vi "sensor model (SubVI).vi"(0 "Sensor noise":bool, 1 "nu in":dbl[](array[numeric])=[-0.0018015758017567245, -0.001192557883344063, -0.016303156939595005, 0.0001609866843798056, -3.986241544768407e-05, 0.002433779794769443], 2 "std HiPAP":dbl=0.1, 3 "Sample period HiPAP":dbl=1000.0, 4 "std IMU":dbl=0.02, 5 "eta in":dbl[](array[numeric])=[0.004584023716384989, -0.00136654983894139, 20.08049813655914, 1.4271590869671887e-05, -0.00011626978763392943, 1.5737394787921046], 6 "Init North":dbl=6971450.0 format="%#.2f", 7 "All Pos mes":bool, 8 "std rad/s":dbl=0.02, 9 "std PG":dbl=0.1, 10 "Seafloor":dbl[](array[numeric])=[30.0, -0.1, 0.0, 0.0, 0.0], 11 "Init East":dbl=395890.0 format="%#.2f", 12 "std DVL":dbl=0.1, 13 "NORTH SHIP":dbl=7100000.0, 14 "HEADING SHIP":dbl=488000.0, 15 "EAST SHIP":dbl=488000.0, 16 "Init Depth":dbl=4.0 format="%#.2f", 17 "std roll&pitch":dbl=0.02) -> (19 "GPS and APOS Strings":string[](array[string]), 20 "COM1":dbl[](array[numeric])=[20.08041093421861, 29.91885735344196, 0.0, 90.0, 2068.0], 23 "COM2":dbl[](array[numeric])=[539999.2486367036, 7200000.006791385, -0.0030178927294211453, -0.0018015758017567245, 12.750414264450102, -85.11865540641482, 20.696406625105084, 54.45747480595215])   [LabVIEW 2014]
uses:
  <vilib>/Analysis/NI_AALBase.lvlib
panel:
  out "Heave":cluster{"Y":dbl[], "Y":dbl[]}[](graph)
  out "Surge":cluster{"Y":dbl[], "Y":dbl[]}[](graph)
  out "Sway":cluster{"Y":dbl[], "Y":dbl[]}[](graph)
  out "PSIMSSB String":string
  out "GPGGA String":string
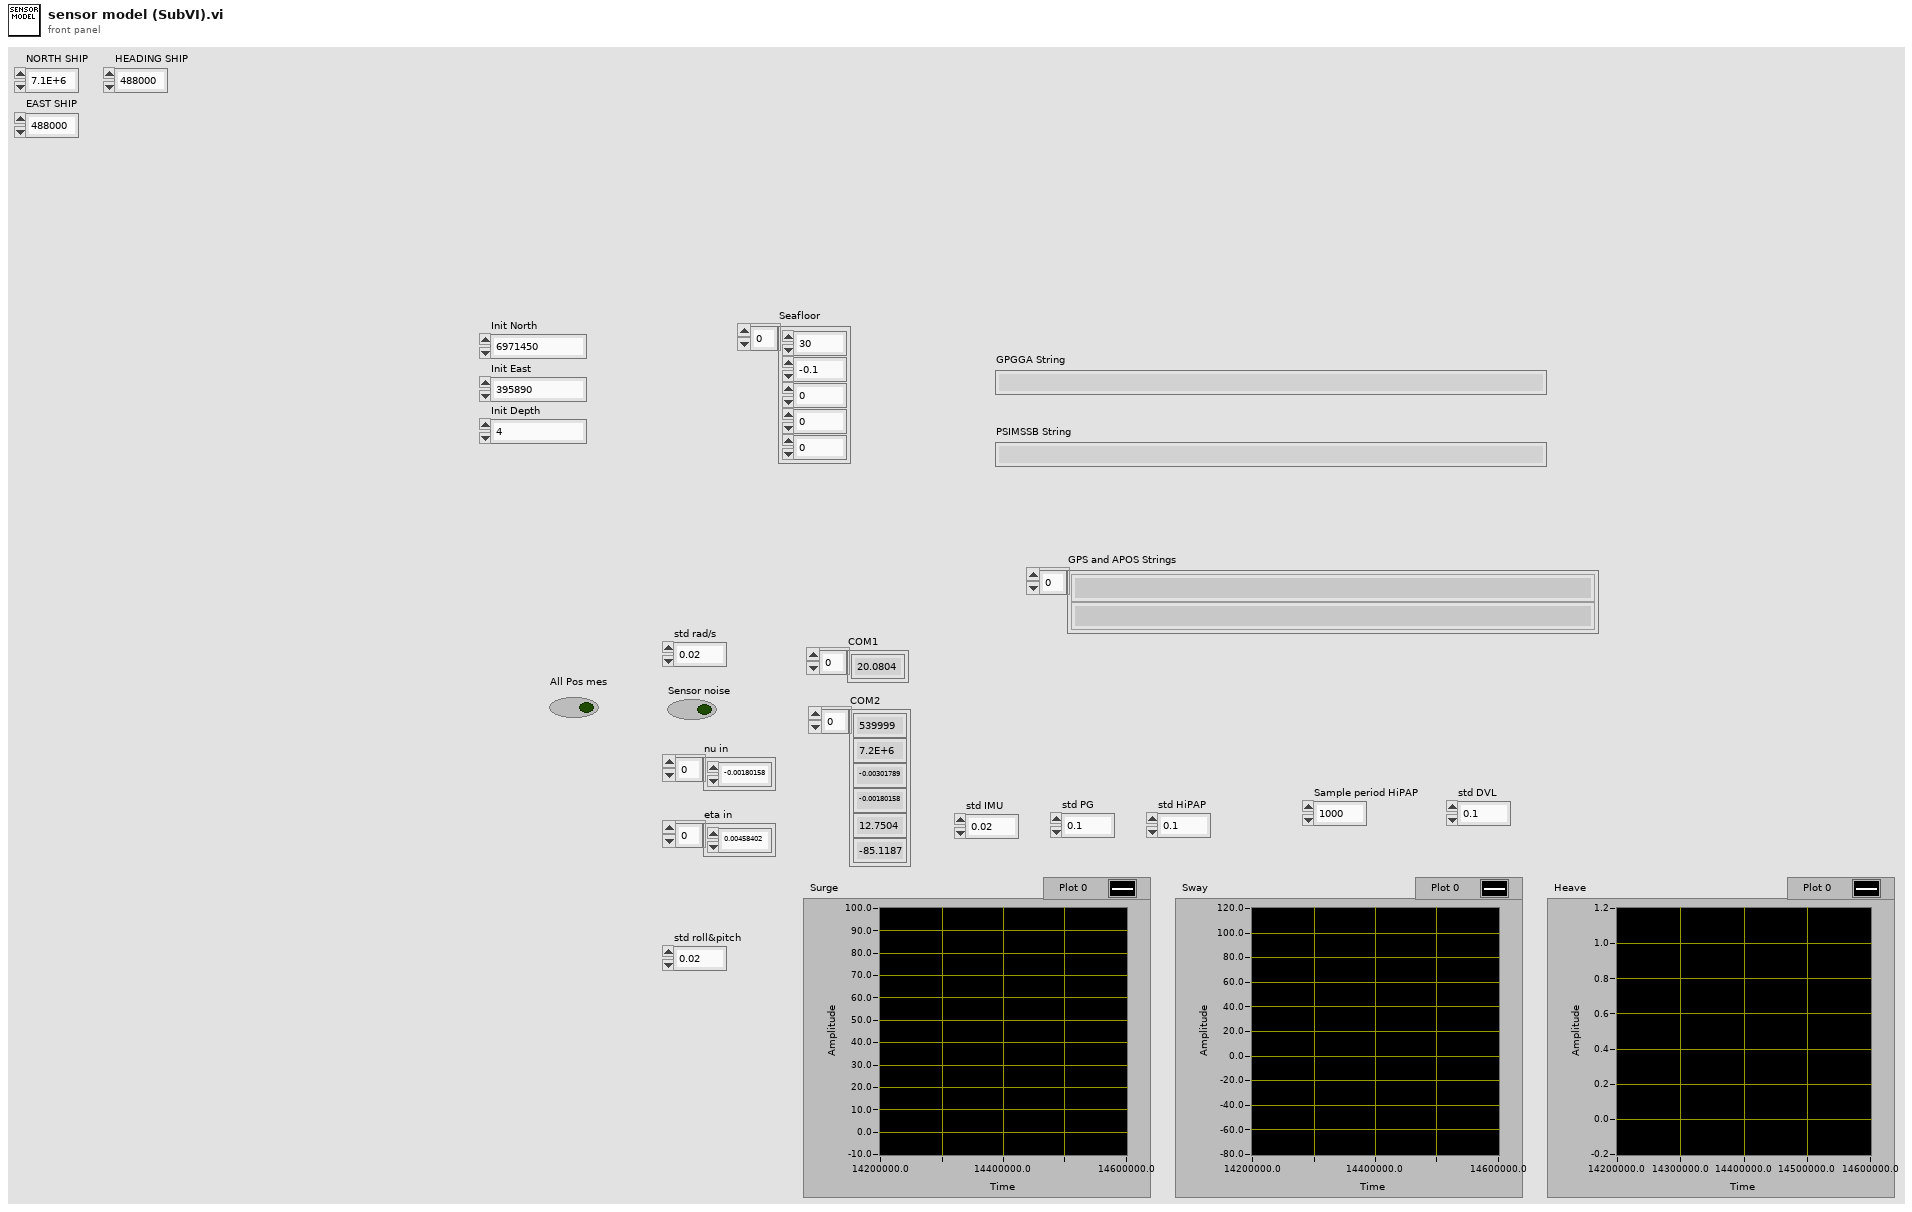
[diagram p1: front panel]
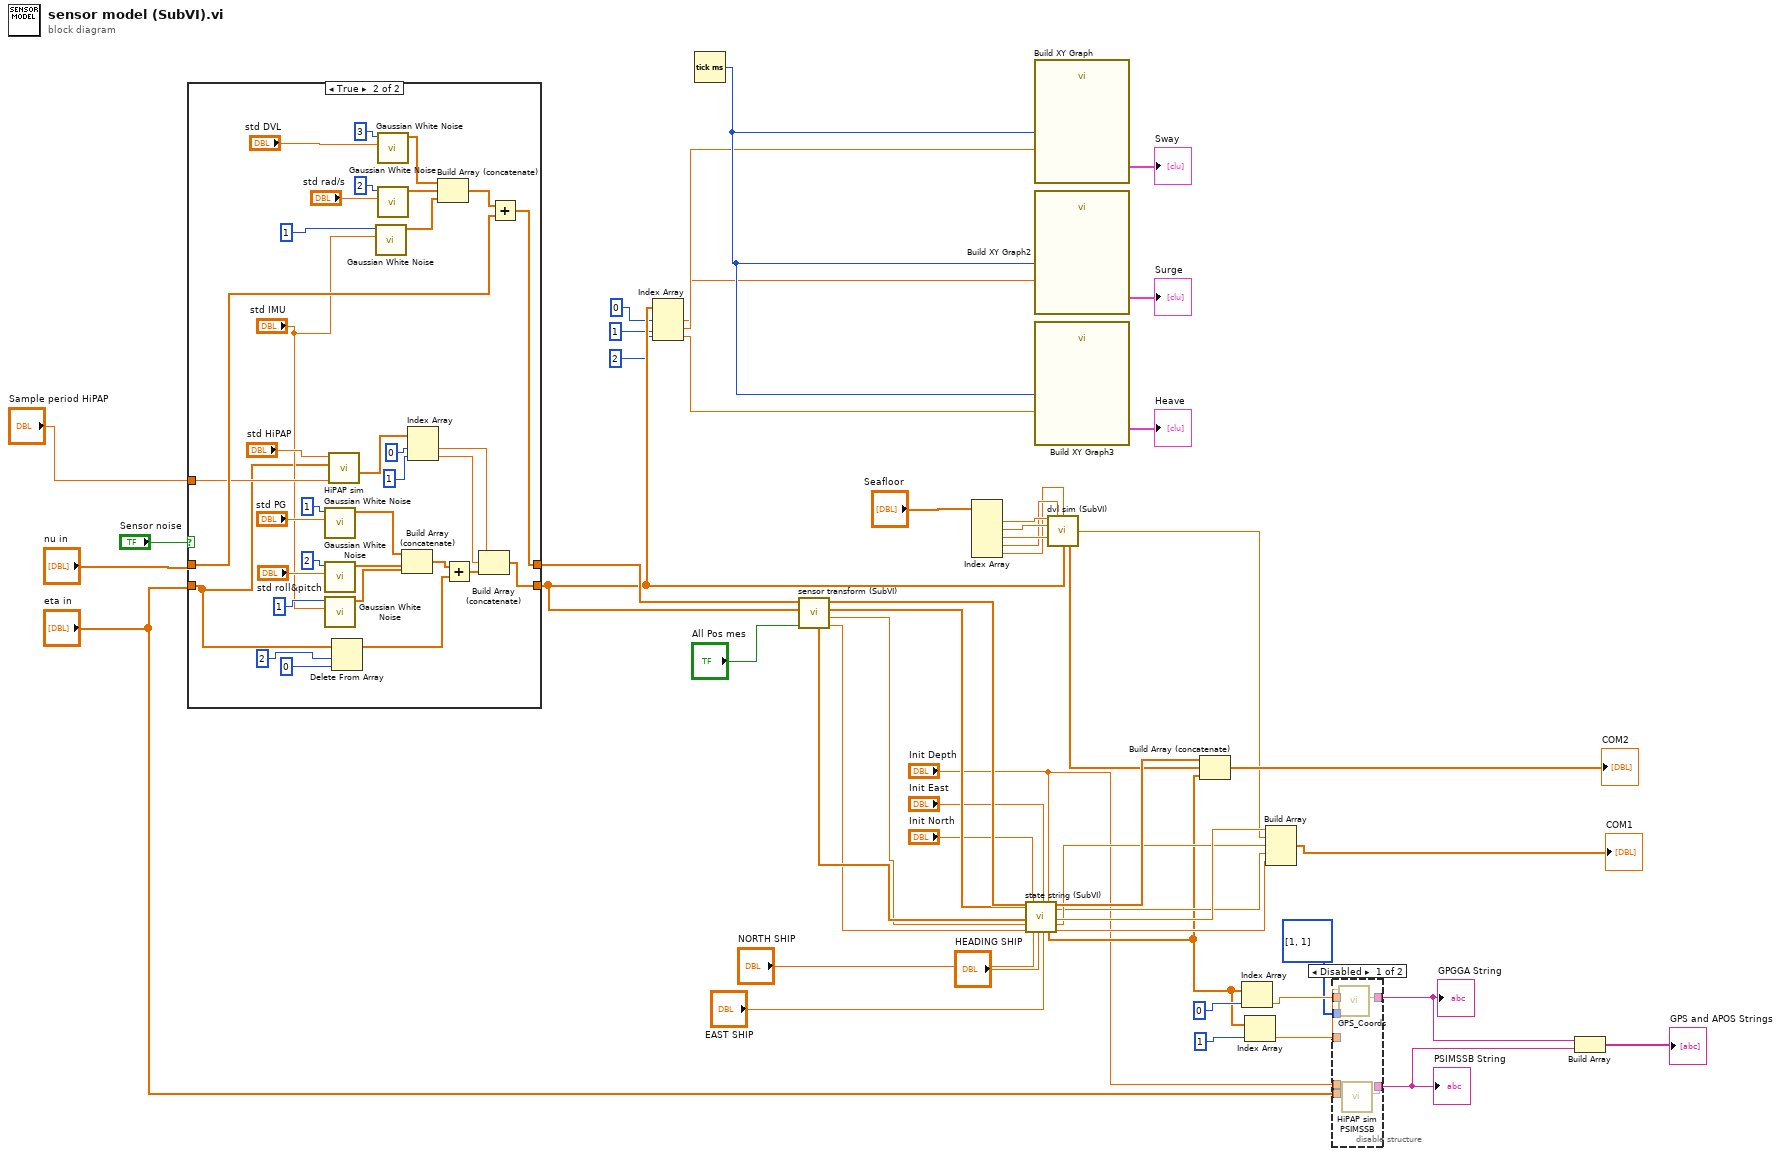
[diagram p0: block diagram]
diagram:
  n1 = case shown="True" "Sensor noise" {
    tunnel: "nu in" -> [w54 w72]
    tunnel: [w54 w74] -> w51
    tunnel: "eta in" -> [w53 w55]
    tunnel: [w53 w64] -> w9
    tunnel: "Sample period HiPAP" -> [_ w71]
    frame False {
    }
    frame True {
      n2 = call <vilib>:"Gaussian White Noise.vi"("standard deviation"="std PG", "samples"=1) -> ("Gaussian noise pattern"=w87:dbl[])  [unwired: 8 in, 1 out]
      n3 = call <vilib>:"Gaussian White Noise.vi"("standard deviation"="std roll&pitch", "samples"=2) -> ("Gaussian noise pattern"=w88:dbl[])  [unwired: 8 in, 1 out]
      n4 = call <vilib>:"Gaussian White Noise.vi"("standard deviation"="std IMU", "samples"=1) -> ("Gaussian noise pattern"=w63:dbl[])  [unwired: 8 in, 1 out]
      n5 = call "HiPAP sim.vi"("Sample period HiPAP (ms)"=w71, "Eta in"=w55, "HiPAP std"="std HiPAP") -> ("Eta out"=w70:dbl[])  [unwired: 8 in]
      n6 = Delete From Array(array=w55, length=2, index=0) -> (array with subset deleted=w56:dbl[])  [unwired: 1 out]
      n7 = call <vilib>:"Gaussian White Noise.vi"("standard deviation"="std IMU", "samples"=1) -> ("Gaussian noise pattern"=w60:dbl[])  [unwired: 8 in, 1 out]
      n8 = call <vilib>:"Gaussian White Noise.vi"("standard deviation"="std DVL", "samples"=3) -> ("Gaussian noise pattern"=w77:dbl[])  [unwired: 8 in, 1 out]
      n9 = call <vilib>:"Gaussian White Noise.vi"("standard deviation"="std rad/s", "samples"=2) -> ("Gaussian noise pattern"=w76:dbl[])  [unwired: 8 in, 1 out]
      n10 = Build Array (concatenate)(w87, w88, w63) -> (w82:dbl[])
      n11 = Index Array(array=w70, index #1=0, index #2=1) -> (element #1=w65:dbl, element #2=w66:dbl)
      n12 = Build Array (concatenate)(w77, w76, w60) -> (w75:dbl[])
      n13 = Add(x=w82, y=w56) -> (x+y=w67:dbl[])
      n14 = Build Array (concatenate)(w65, w66, w67) -> (w64:dbl[])
      n15 = Add(x=w75, y=w72) -> (x+y=w74:dbl[])
    }
  }
  n16 = Index Array(array=w9, index #1=0, index #2=1, index #3=2) -> (element #1=w2:dbl, element #2=w3:dbl, element #3=w4:dbl)
  n17 = Tick Count (ms)() -> (millisecond timer value=w5:u32)
  n18 = call "sensor transform (SubVI).vi"("All Pos mes"="All Pos mes", "eta"=w9, "nu"=w51) -> ("C_out"=w40:dbl, "PG_out"=w41:dbl, "DVL_out"=w43:dbl[], "TP_out"=w44:dbl[], "IMU_out"=w42:dbl[])  [unwired: 4 in]
  n19 = Index Array(array="Seafloor") -> (element #1=w49:dbl, element #2=w48:dbl, element #3=w47:dbl, element #4=w46:dbl, element #5=w45:dbl)  [unwired: 5 in]
  n20 = call "state string (SubVI).vi"("TP_in"=w44, "DVL_in"=w43, "IMU_in"=w42, "PG_in"=w41, "C_in"=w40, "Init North"="Init North", "NORTH SHIP"="NORTH SHIP", "HEADING SHIP"="HEADING SHIP", "Init East"="Init East", "EAST SHIP"="EAST SHIP", "Init Depth"="Init Depth") -> ("Ship_pos"=w22:dbl[], "TP_DVL"=w39:dbl[], "psi"=w33:dbl, "depth"=w36:dbl, "turns"=w34:dbl, "r [counts]"=w32:dbl)  [unwired: 3 in]
  n21 = call "Build XY Graph"("Y Input"=w3, "X Input"=w5) -> ("XY Graph"=→"Sway":cluster{"Y":dbl[], "Y":dbl[]}[])  [unwired: 3 in, 6 out]
  n22 = call "Build XY Graph2"("Y Input"=w2, "X Input"=w5) -> ("XY Graph"=→"Surge":cluster{"Y":dbl[], "Y":dbl[]}[])  [unwired: 3 in, 6 out]
  n23 = call "Build XY Graph3"("Y Input"=w4, "X Input"=w5) -> ("XY Graph"=→"Heave":cluster{"Y":dbl[], "Y":dbl[]}[])  [unwired: 3 in, 6 out]
  n24 = call "dvl sim (SubVI).vi"("IC_Water_depth"=w49, "a2"=w46, "b2"=w45, "a1"=w48, "b1"=w47, "eta"=w9) -> ("alt"=w35:dbl, "DVL_alts"=w38:dbl[])  [unwired: 3 in, 5 out]
  n25 = Build Array (concatenate)(w39, w38, w22) -> (→"COM2":dbl[])
  n26 = Index Array(array=w22, index=0) -> (element=w23:dbl)
  n27 = Index Array(array=w22, index=1) -> (element=w20:dbl)
  n28 = Build Array(w36, w35, w34, w33, w32) -> (→"COM1":dbl[])
  n29 = disable-structure shown="Disabled" {
    disable-tunnel: w23 -> [w95 _]
    disable-tunnel: w20 -> [w94 _]
    disable-tunnel: [w93 _] -> w18
    disable-tunnel: [w92 _] -> w17
    disable-tunnel: "Init Depth" -> [w91 _]
    disable-tunnel: i32[] [1, 1] -> [w90 _]
    disable-tunnel: "eta in" -> [w89 _]
    frame Disabled {
      n30 = call "GPS_Coords.vi"("Ship Movement (meters)"=w90, "Ship North Pos (UTM)"=w95, "Ship East Pos (UTM)"=w94) -> ("$GPGGA string"=w93:string)  [unwired: 8 in]
      n31 = call "HiPAP sim PSIMSSB.vi"("Eta in"=w89, "Init Depth"=w91) -> ("PSIMSSB String"=w92:string)  [unwired: 9 in]
    }
    frame Enabled {
    }
  }
  "GPGGA String" <- w18
  "PSIMSSB String" <- w17
  n32 = Build Array(w18, w17) -> (→"GPS and APOS Strings":string[])
